vi "Main.vi"(8 "error in (no error)":errorcluster, 11 "AutofocusBase in":refnum<class "Autofocus.lvclass">) -> (0 "error out":errorcluster, 3 "component":refnum<class "Autofocus.lvclass">)   [LabVIEW 2012, in "Autofocus.lvclass"]
doc: "Main VI of the component."
uses:
  Autofocus.lvclass
  <vilib>/Distrio/Murmex/Murmex/command_enum.ctl
  ROI size.ctl
  Sharpness Measure.ctl
  Search algorithm.ctl
  <vilib>/Distrio/Murmex/InitialiseMessage/InitialiseMessage.lvclass
  <vilib>/Distrio/Murmex/Murmex/update_cluster.ctl
  <vilib>/Distrio/Murmex/TerminateMessage/TerminateMessage.lvclass
  <vilib>/Distrio/Murmex/StopMessage/StopMessage.lvclass
  <vilib>/Distrio/Murmex/ConfigureMessage/ConfigureMessage.lvclass
  <vilib>/Distrio/Murmex/Murmex/Set configure at initialise.vi
  <vilib>/Distrio/Murmex/Murmex/Set log reference.vi
  <vilib>/Distrio/Murmex/Murmex/Set VI reference.vi
  <vilib>/Distrio/Murmex/Murmex/Get ID.vi
  <vilib>/Distrio/Murmex/Murmex/Murmex.lvclass
  <vilib>/Distrio/Murmex/Message/Message.lvclass
panel:
  out "terminate?":bool=TRUE
  in  "button::stop":bool
  in  "button::quit":bool
  in  "Tab Control":enum32{"User", "Debug"}(tab)
  out "Focus curve":cluster{"x array":dbl[], "y array":dbl[]}(graph)
  in  "Search Algorithm":T1
  in  "Sharpness measure":T2
  in  "ROI size":T3 items=["50x50"=50, "100x100"=100, "250x250"=250]
  in  "Region sampling":bool
  in  "button::configure":bool
  in  "button::send":bool
  in  "ID":string="stage"
  in  "command":T4
  in  "Generic command":string
  out "log":string
  # "Region sampling"
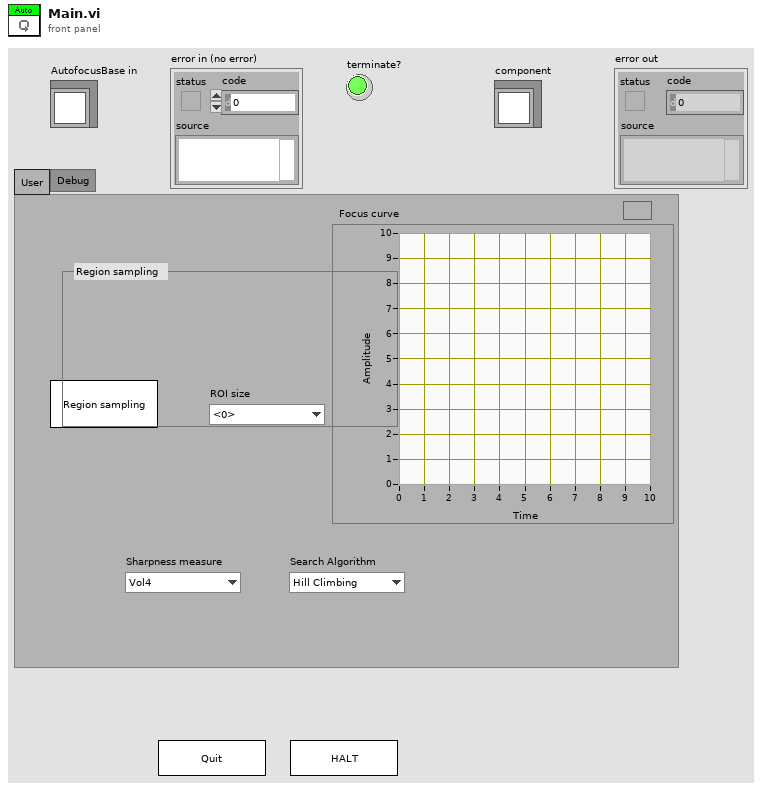
[diagram p1: front panel]
types:
  T1 = typedef "Autofocus.lvclass/Search algorithm.ctl" = enum16{"Hill Climbing"}
  T2 = typedef "Autofocus.lvclass/Sharpness Measure.ctl" = enum16{"Vol4", "Gradient Square"}
  T3 = typedef "Autofocus.lvclass/ROI size.ctl" = u16
  T4 = typedef "Murmex.lvlib/Murmex.lvclass/command_enum.ctl" = enum16{"null", "initialise", "reset", "terminate", "acknowledge", "update", "inspect", "inform", "proceed", "start", "stop", "fetch", "configure", "generic"}
  T5 = enum8{"Enabled", "Disabled", "Disabled and Grayed Out"}
  T6 = typedef "Murmex.lvlib/Murmex.lvclass/update_cluster.ctl" = cluster{"target ID":string, "key chains":string[], "values":variant[]}
  T7 = typedef "Murmex.lvlib/Murmex.lvclass/Event type enumerations.ctl" = enum16{"before", "after"}
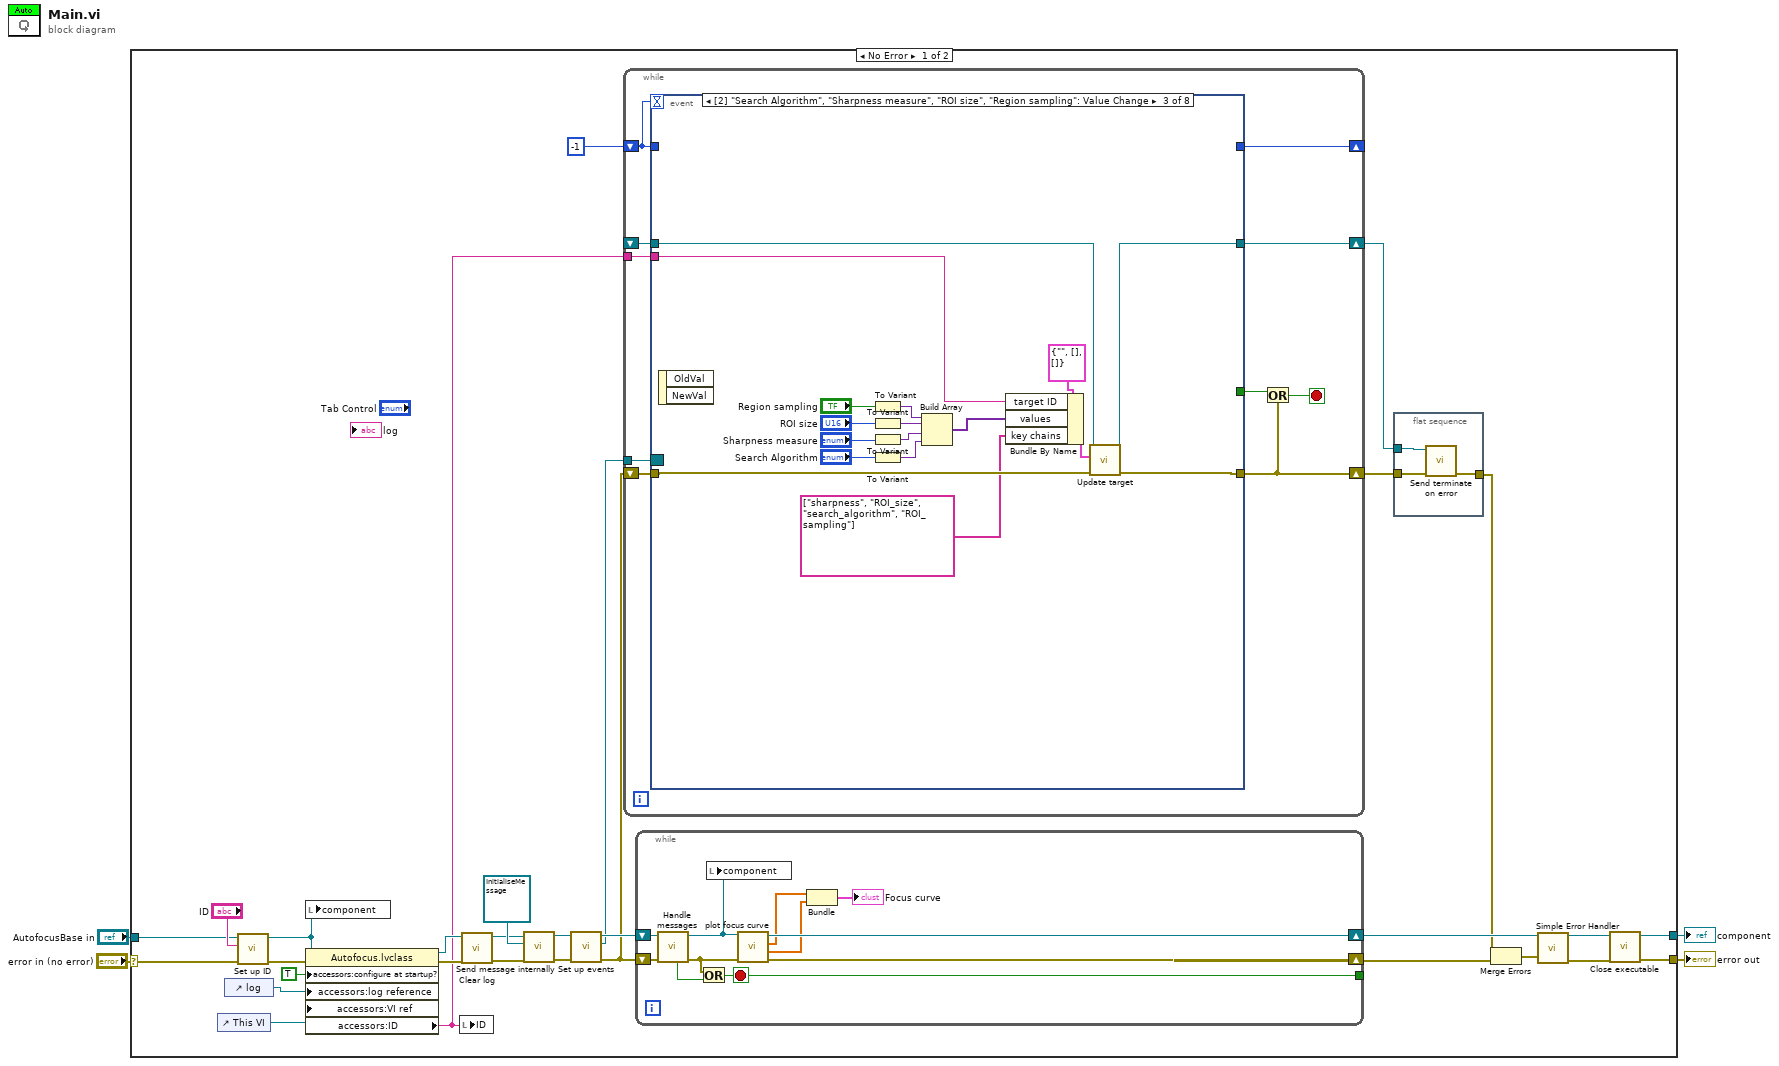
[diagram p0: block diagram]
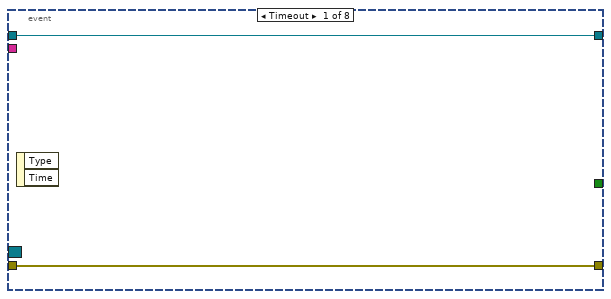
[diagram p2: hidden frame]
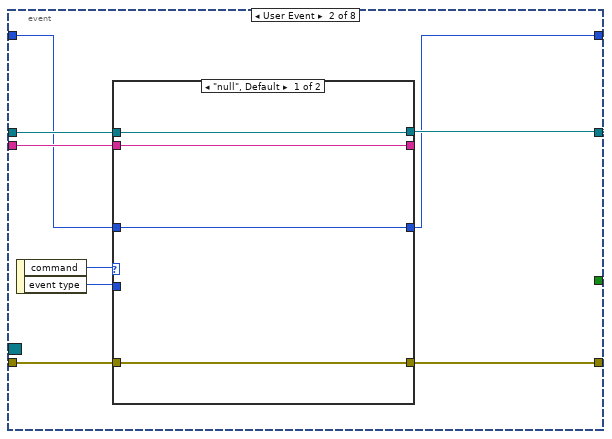
[diagram p3: hidden frame]
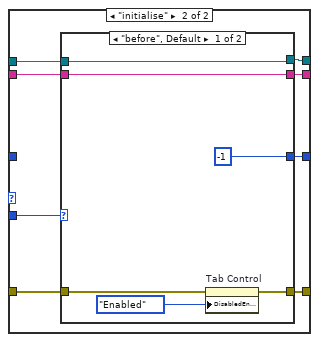
[diagram p4: hidden frame]
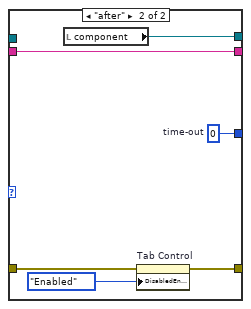
[diagram p5: hidden frame]
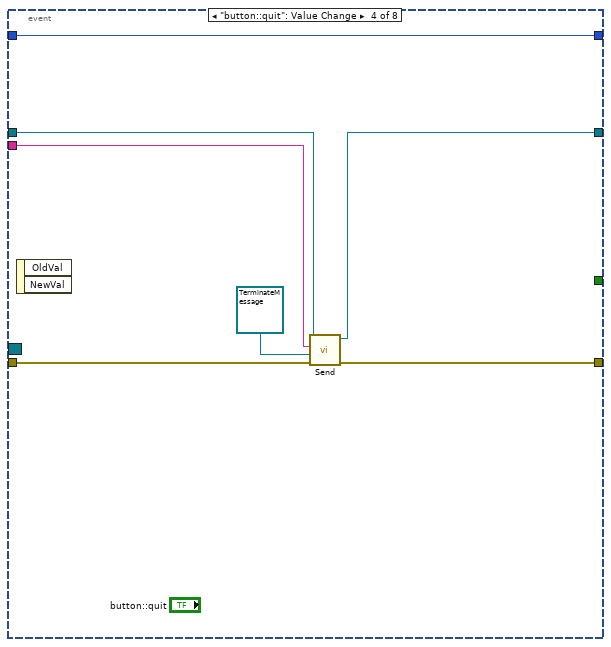
[diagram p6: hidden frame]
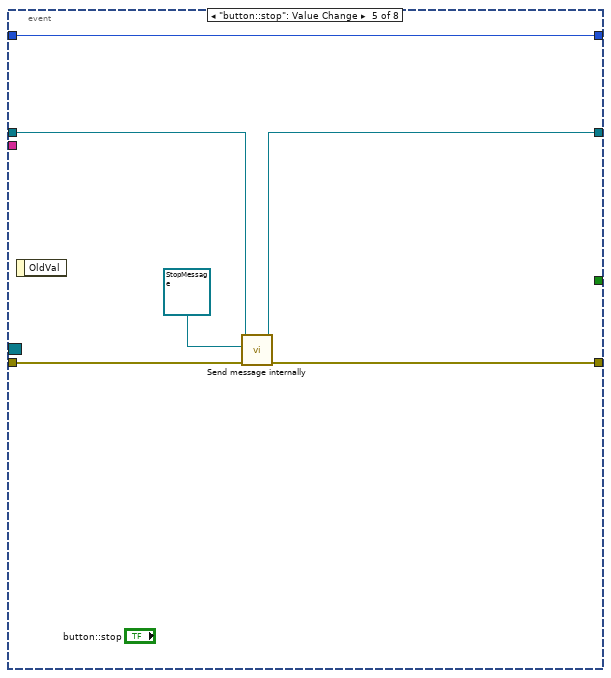
[diagram p7: hidden frame]
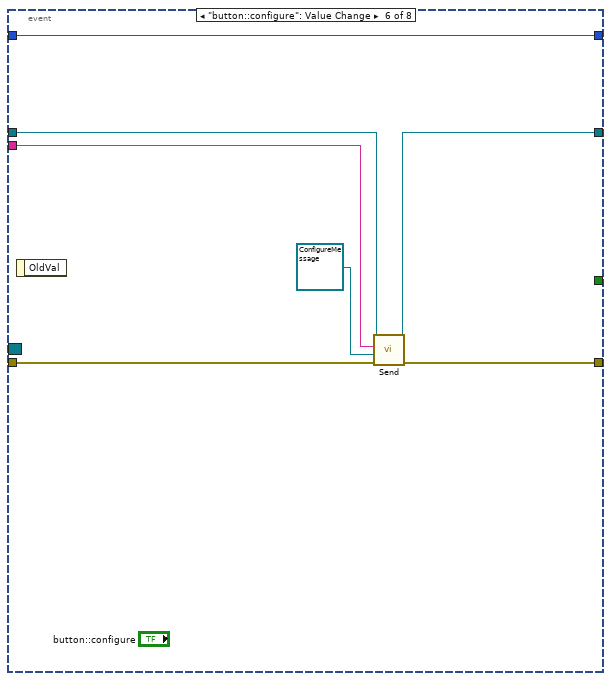
[diagram p8: hidden frame]
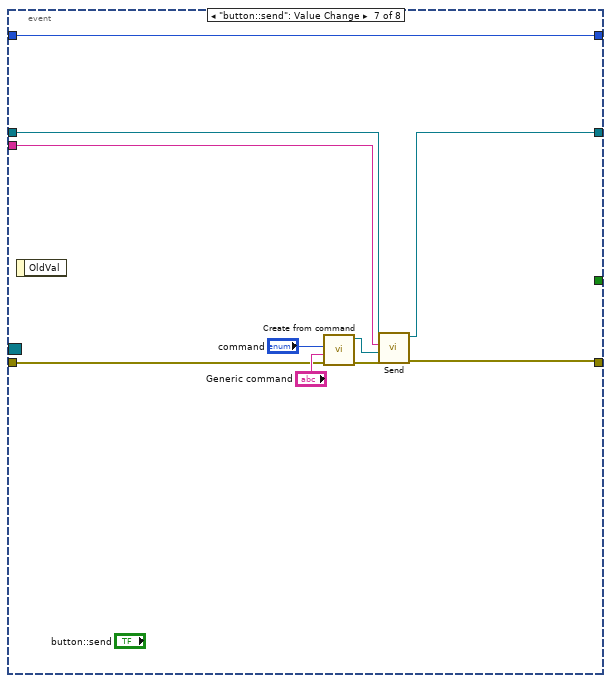
[diagram p9: hidden frame]
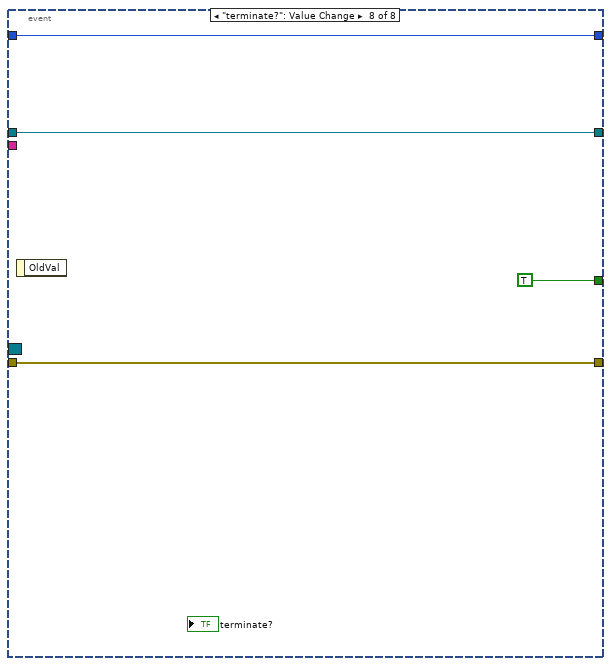
[diagram p10: hidden frame]
diagram:
  n1 = case shown="No Error" "error in (no error)" {
    selector: "error in (no error)" -> [w31 w145]
    tunnel: "AutofocusBase in" -> [w32 w144]
    tunnel: [w9 w145] -> w2
    tunnel: [w8 w144] -> w1
    frame No Error {
      n2 = control-ref of="This VI"() -> (w28:refnum<vi>)
      n3 = control-ref of="log"() -> (w10:refnum<vi>)
      n4 = call <vilib>:"Set up ID.vi"("error in (no error)"=w31, "component ID"="ID", "MurmexBase in"=w32) -> ("error out"=w30:errorcluster, "MurmexBase out"=w20:refnum<class "Autofocus.lvclass">)  [unwired: 6 in, 1 out]
      n5 = local write "component"(w20) -> ()
      n6 = property class="Autofocus.lvclass"(reference=w20, error in=w30, "accessors:configure at startup?"=TRUE ("configure at startup?"), "accessors:log reference"=w10, "accessors:VI ref"=w28) -> (reference out=w21:refnum<class "Autofocus.lvclass">, error out=w22:errorcluster, "accessors:ID"=w11:string)
      n7 = local write "ID"(w11) -> ()
      n8 = call <vilib>:"Clear log.vi"("error in (no error)"=w22, "MurmexBase in"=w21) -> ("error out"=w23:errorcluster, "MurmexBase out"=w24:refnum<class "Autofocus.lvclass">)  [unwired: 8 in]
      n9 = call <vilib>:"Send message internally.vi"("error in (no error)"=w23, "Message"=refnum<class "InitialiseMessage.lvclass"> refnum ("Distrio Murmex 1.1:InitialiseMessage"), "Murmex in"=w24) -> ("error out"=w26:errorcluster, "Murmex out"=w27:refnum<class "Autofocus.lvclass">)  [unwired: 7 in]
      n10 = call <vilib>:"Set up events.vi"("error in (no error)"=w26, "MurmexBase in"=w27) -> ("error out"=w13:errorcluster, "Event Registration Refnum"=w14:refnum<event-registration>, "MurmexBase out"=w19:refnum<class "Autofocus.lvclass">)  [unwired: 7 in]
      n11 = while {
        tunnel: w14 -> [w46]
        shift-right: [w38] -> w6
        shift-left: w13 -> [w45]
        shift-right: [w40] -> _
        shift-left: -1 -> [w44]
        tunnel: w11 -> [w43]
        shift-right: [w42] -> w7
        shift-left: _ -> [w41]
        stop <- w37 stop-if-true
        n12 = event shown="[2] \"Search Algorithm\", \"Sharpness measure\", \"ROI size\", \"Region sampling\": Value Change" {
          selector: w46 -> [_ _ _ _ _ _ _ _]
          dyn-events: _ -> [_ _ _ _ _ _ _ _]
          timeout: w44 -> [_ _ _ _ _ _ _ _]
          tunnel: w45 -> [w48 w57 w92 w104 w110 w117 w124 w132]
          tunnel: w44 -> [_ w49 _ w99 w106 w112 w119 w129]
          tunnel: w43 -> [_ w56 w85 w102 _ w113 w120 _]
          tunnel: [w47 w53 w83 w100 w107 w114 w121 w130] -> w42
          tunnel: w41 -> [w47 w52 w84 w101 w108 w115 w122 w130]
          tunnel: [_ w51 _ w99 w106 w112 w119 w129] -> w40
          tunnel: [w48 w50 w91 w103 w109 w116 w123 w132] -> w38
          tunnel: [_ _ _ _ _ _ _ TRUE] -> w39
          event Timeout {
            n13 = event-data() -> ()  [unwired: 1 in, 2 out]
          }
          event User Event {
            n14 = event-data() -> ("command"=w55:T4, "event type"=w54:T7)  [unwired: 1 in]
            n15 = case shown="\"null\", Default" w55 {
              tunnel: w57 -> [w60 w69]
              tunnel: [w60 w68] -> w50
              tunnel: w56 -> [w61 w67]
              tunnel: [w58 w66] -> w53
              tunnel: [w61 w65] -> _
              tunnel: w54 -> [_ w64]
              tunnel: [w59 w63] -> w51
              tunnel: w52 -> [w58 w62]
              tunnel: w49 -> [w59 _]
              frame "null", Default {
              }
              frame "initialise" {
                n16 = case shown="\"before\", Default" w64 {
                  tunnel: [w74 w80] -> w68
                  tunnel: w69 -> [w75 w81]
                  tunnel: w67 -> [w72 w77]
                  tunnel: [w70 w79] -> w66
                  tunnel: [w72 w77] -> w65
                  tunnel: [-1 w76] -> w63
                  tunnel: w62 -> [w70 _]
                  frame "before", Default {
                    n17 = property on="Tab Control" class="TabCtl (strict)"(error in=w75, "DisabledEnum"=T5."Enabled" ("Disabled")) -> (error out=w74:errorcluster)  [unwired: 1 in, 1 out]
                  }
                  frame "after" {
                    w76 = 0  # time-out
                    n18 = local read "component"() -> (w79:refnum<class "Autofocus.lvclass">)
                    n19 = property on="Tab Control" class="TabCtl (strict)"(error in=w81, "DisabledEnum"=T5."Enabled" ("Disabled")) -> (error out=w80:errorcluster)  [unwired: 1 in, 1 out]
                  }
                }
              }
            }
          }
          event "Region sampling": Value Change {
            n20 = event-data() -> ()  [unwired: 1 in, 2 out]
            n21 = To Variant(anything="Region sampling") -> (Variant=w96:variant)
            n22 = To Variant(anything="ROI size") -> (Variant=w95:variant)
            n23 = To Variant(anything="Sharpness measure") -> (Variant=w94:variant)
            n24 = To Variant(anything="Search Algorithm") -> (Variant=w90:variant)
            n25 = Build Array(w96, w95, w94, w90) -> (w93:variant[])
            n26 = Bundle By Name(cluster=T6 {"target ID"="", "key chains"=[], "values"=[]} ("update cluster"), "target ID"=w85, "values"=w93, "key chains"=string[] ["sharpness", "ROI_size", "search_algorithm", "ROI_sampling"]) -> (w98:T6)
            n27 = call <vilib>:"Update target.vi"("error in (no error)"=w92, "update cluster"=w98, "MurmexBase in"=w84) -> ("error out"=w91:errorcluster, "MurmexBase out"=w83:refnum<class "Autofocus.lvclass">)  [unwired: 7 in]
          }
          event "button::quit": Value Change {
            n28 = event-data() -> ()  [unwired: 1 in, 2 out]
            n29 = call <vilib>:"Send.vi"("error in (no error)"=w104, "Message"=refnum<class "TerminateMessage.lvclass"> refnum ("Murmex.lvlib:TerminateMessage"), "recipient"=w102, "Murmex in"=w101) -> ("error out"=w103:errorcluster, "Murmex out"=w100:refnum<class "Autofocus.lvclass">)  [unwired: 6 in]
          }
          event "button::stop": Value Change {
            n30 = event-data() -> ()  [unwired: 1 in, 1 out]
            n31 = call <vilib>:"Send message internally.vi"("error in (no error)"=w110, "Message"=refnum<class "StopMessage.lvclass"> refnum ("Distrio Murmex 1.5:StopMessage"), "Murmex in"=w108) -> ("error out"=w109:errorcluster, "Murmex out"=w107:refnum<class "Autofocus.lvclass">)  [unwired: 7 in]
          }
          event "button::configure": Value Change {
            n32 = event-data() -> ()  [unwired: 1 in, 1 out]
            n33 = call <vilib>:"Send.vi"("error in (no error)"=w117, "Message"=refnum<class "ConfigureMessage.lvclass"> refnum ("Distrio Murmex 1.1:ConfigureMessage"), "recipient"=w113, "Murmex in"=w115) -> ("error out"=w116:errorcluster, "Murmex out"=w114:refnum<class "Autofocus.lvclass">)  [unwired: 6 in]
          }
          event "button::send": Value Change {
            n34 = event-data() -> ()  [unwired: 1 in, 1 out]
            n35 = call <vilib>:"Create from command.vi"("error in (no error)"=w124, "generic command"="Generic command", "command"="command") -> ("error out"=w127:errorcluster, "Message out"=w126:refnum<class "Message.lvclass">)  [unwired: 7 in]
            n36 = call <vilib>:"Send.vi"("error in (no error)"=w127, "Message"=w126, "recipient"=w120, "Murmex in"=w122) -> ("error out"=w123:errorcluster, "Murmex out"=w121:refnum<class "Autofocus.lvclass">)  [unwired: 6 in]
          }
          event "terminate?": Value Change {
            n37 = event-data() -> ()  [unwired: 1 in, 1 out]
          }
        }
        n38 = Or(x=w39, y=w38) -> (x .or. y?=w37:bool)
      }
      n39 = while {
        shift-right: [w137] -> w15
        shift-left: w19 -> [w142]
        shift-right: [w135] -> w16
        shift-left: w13 -> [w143]
        tunnel: [w140] -> _
        stop <- w140 stop-if-true
        n40 = call <vilib>:"Handle messages.vi"("error in (no error)"=w143, "Murmex in"=w142) -> ("error out"=w136:errorcluster, "Murmex out"=w138:refnum<class "Autofocus.lvclass">, "terminated?"=w141:bool)  [unwired: 7 in]
        n41 = Or(x=w136, y=w141) -> (x .or. y?=w140:bool)
        n42 = local write "component"(w138) -> ()
        n43 = call-dynamic "plot focus curve.vi"("error in (no error)"=w136, "Autofocus in"=w138) -> ("error out"=w135:errorcluster, "x array"=w133:dbl[], "y array"=w134:dbl[], "Autofocus out"=w137:refnum<class "Autofocus.lvclass">)  [unwired: 6 in]
        n44 = Bundle("y array"=w134, "x array"=w133) -> (→"Focus curve":cluster{"y array":dbl[], "x array":dbl[]})  [unwired: 1 in]
      }
      n45 = flat-sequence {
        tunnel: w6 -> [w36]
        tunnel: [w35] -> w5
        tunnel: w7 -> [w34]
        frame #0 {
          n46 = call <vilib>:"Send terminate on error.vi"("error in (no error)"=w36, "Murmex in"=w34) -> ("error out"=w35:errorcluster)  [unwired: 8 in, 1 out]
        }
      }
      n47 = Merge Errors(w5, w16) -> (w17:errorcluster)
      n48 = call <vilib>:"Simple Error Handler.vi"("error in (no error)"=w17) -> ("error out"=w18:errorcluster)  [unwired: 4 in, 4 out]
      n49 = call <vilib>:"Close executable.vi"("error in (no error)"=w18, "MurmexBase in"=w15) -> ("error out"=w9:errorcluster, "MurmexBase out"=w8:refnum<class "Autofocus.lvclass">)  [unwired: 8 in]
    }
    frame Error {
    }
  }
  "error out" <- w2
  "component" <- w1
